vi "Config Data Type.vi"(8 "error in (no error)":errorcluster, 11 "Group in":refnum<class "Group.lvclass">) -> (0 "error out":errorcluster, 2 "Group Data Type":T1, 3 "Group out":refnum<class "Group.lvclass">)   [LabVIEW 2020, in "Vecto.lvlib" / "Group.lvclass"]
uses:
  Group.lvclass
  Group Config/Group Config.lvclass
  Group Data Type.ctl
  VectoConfig/VectoConfig.lvlib
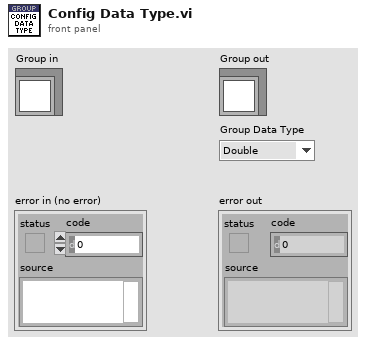
[diagram p1: front panel]
types:
  T1 = typedef "VectoConfig.lvlib/Group Data Type.ctl" = enum16{"Double", "String", "Bool"}
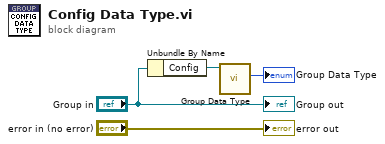
[diagram p0: block diagram]
diagram:
  n1 = Unbundle By Name("Group in") -> ("Config"=w4:refnum<class "Group Config.lvclass">)
  n2 = call "Group Data Type.vi"("Group Config in"=w4) -> ("Data Type"=→"Group Data Type":T1)  [unwired: 8 in, 2 out]
  "error out" <- "error in (no error)"
  "Group out" <- "Group in"
